vi "Gray2Num.vi"() -> ()   [LabVIEW 2018]
panel:
  out "Decimal Code":u32
  out "Output(Binery Code)":bool[](array[boolean])
  in  "Input(Gray code)":bool[](array[boolean])
  # "bit Low"
  # "bit High"
  # "bit Low"
  # "bit High"
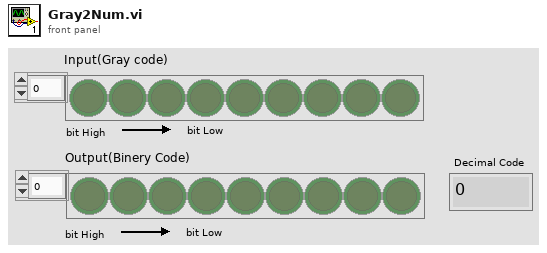
[diagram p1: front panel]
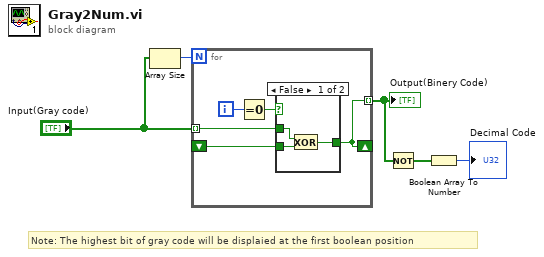
[diagram p0: block diagram]
diagram:
  # "Note: The highest bit of gray code will be displaied at the first boolean position"
  n1 = Array Size(array="Input(Gray code)") -> (size(s)=w5:i32)
  n2 = for {
    N: w5 -> [_]
    tunnel: "Input(Gray code)" -> [w6] mode=indexing
    shift-right: [w7] -> _
    shift-left: _ -> [w8]
    tunnel: [w7] -> w1 mode=indexing
    i -> [w10]
    n3 = Equal To 0?(x=w10) -> (x = 0?=w9:bool)
    n4 = case shown="False" w9 {
      tunnel: [w13 w14] -> w7
      tunnel: w8 -> [w12 _]
      tunnel: w6 -> [w11 w14]
      frame False {
        n5 = Exclusive Or(1:w12, 2:w11) -> (0:w13:bool)
      }
      frame True {
      }
    }
  }
  "Output(Binery Code)" <- w1
  n6 = Not(x=w1) -> (.not. x?=w2:bool[])
  n7 = Boolean Array To Number(Boolean array=w2) -> (number=→"Decimal Code":u32)
